vi "SingleFitDoubleExponential.vi"(0 "Scan rate (Hz)":dbl, 5 "Last point to average for baseline":i32=5, 9 "Input decay":dbl[](array[numeric]), 11 "Input Variance":dbl[](array[numeric])) -> (3 "mean and fit":dbl[][](graph), 4 "amplitude":dbl=1.3790672561842066 caption="Amplitude (au)" format="%#_3g", 6 "Standard error Amplitude":dbl=8.774972224805227 format="%#_3g", 8 "Area (au)":dbl=8.774972224805227 format="%#_3g", 10 "Residu (au)":dbl=8.774972224805227 format="%#_3g", 14 "Standard error Tau (us)":dbl=8.774972224805227 format="%#_3g", 15 "Tau (us)":dbl=8.774972224805227 format="%#_3g")   [LabVIEW 2013]
uses:
  <vilib>/Analysis/baseanly.llb/Mean (DBL).vi
  <vilib>/gmath/NumericalOptimization/Nonlinear Curve Fit LM formula string.vi
  <vilib>/gmath/NI_Gmath.lvlib
  <vilib>/Analysis/NI_AALBase.lvlib
panel:
  out "stdev a1":dbl
  out "a1":dbl
  out "Input DecaySize":dbl
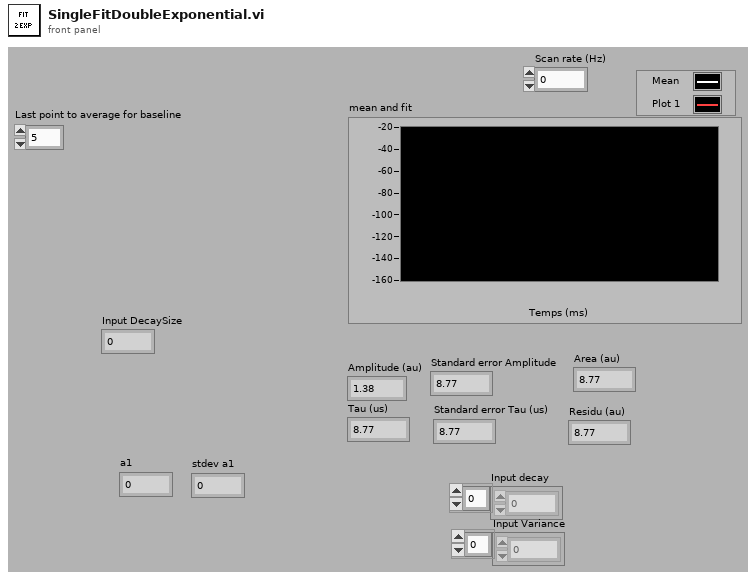
[diagram p1: front panel]
types:
  T1 = cluster{"model":string, "Parameters":string[], "x":string}
  T2 = typedef "NI_Matrix.lvlib/RealMatrix.ctl" = dbl[][]
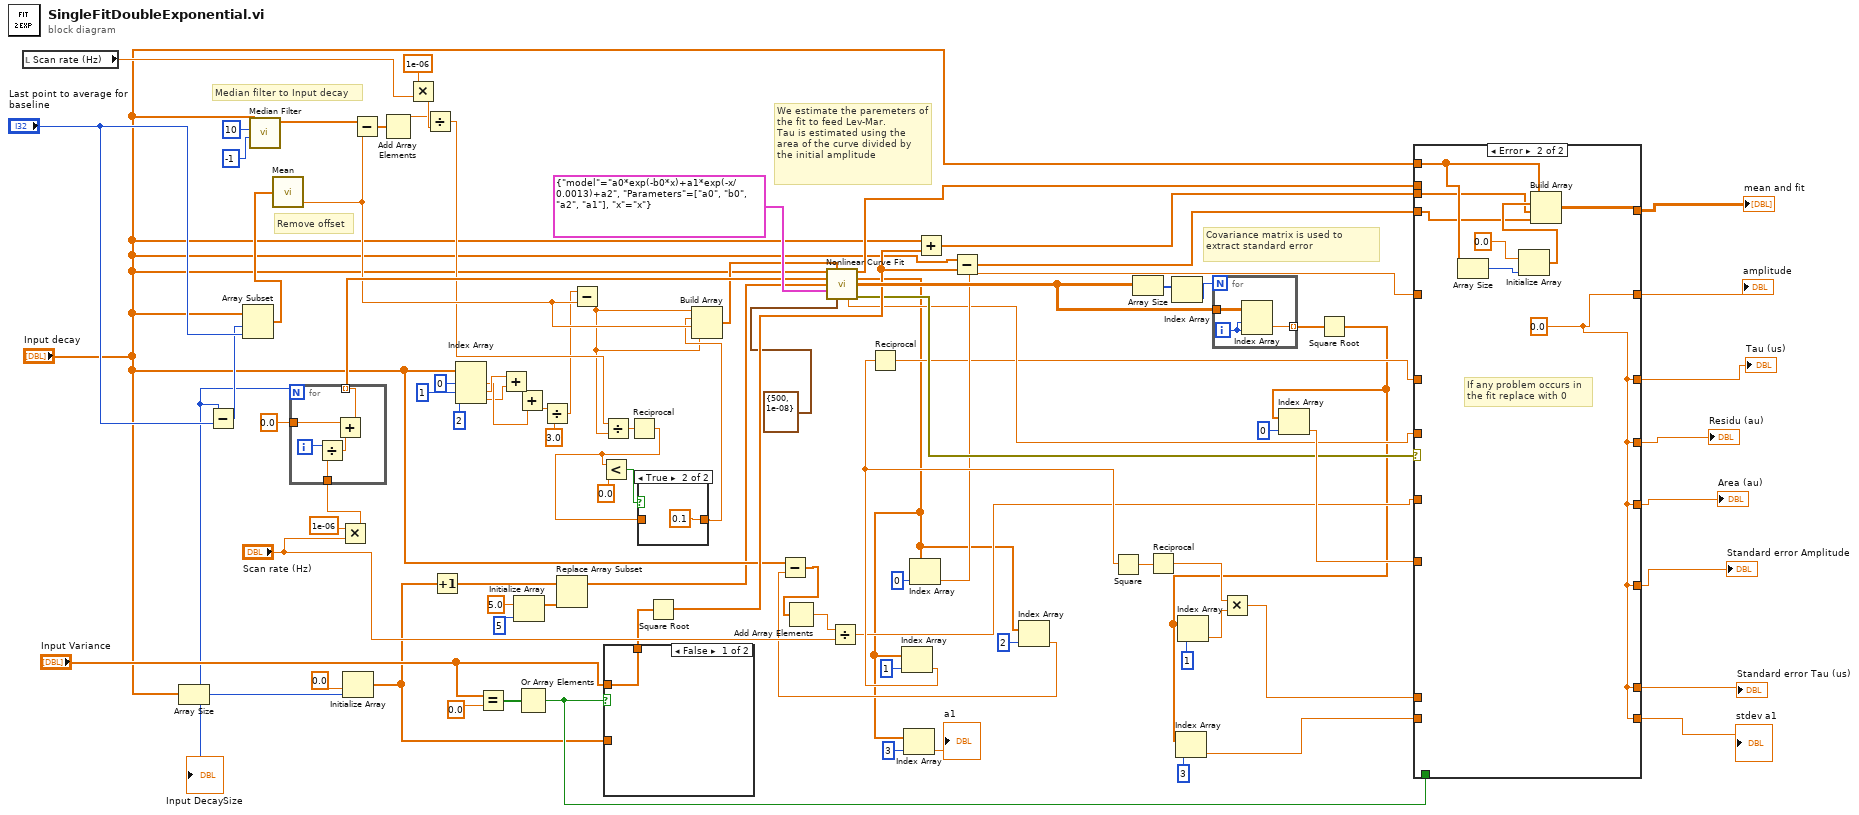
[diagram p0: block diagram]
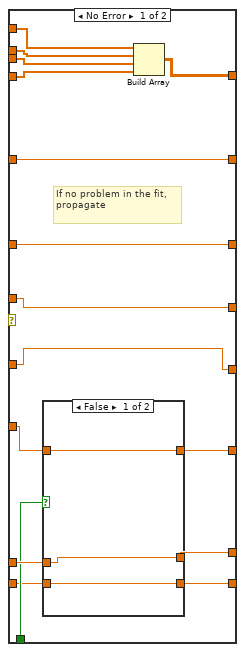
[diagram p3: hidden frame]
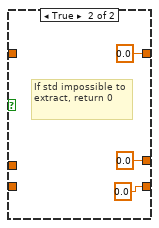
[diagram p4: hidden frame]
diagram:
  # "Median filter to Input decay"
  # "Covariance matrix is used to extract standard error"
  # "Remove offset"
  # "We estimate the paremeters of the fit to feed Lev-Mar.\nTau is estimated using the area of the curve divided by the initial amplitude"
  n1 = local read "Scan rate (Hz)"() -> (w76:dbl)
  n2 = Array Size(array="Input decay") -> (size(s)=w26:i32)
  "Input DecaySize" <- w26
  n3 = Subtract(x=w26, y="Last point to average for baseline") -> (x-y=w91:i32)
  n4 = Array Subset(array="Input decay", index=w91, length="Last point to average for baseline") -> (w90:dbl[])
  n5 = call <vilib>:"Median Filter.vi"("right rank"=-1, "left rank"=10, "X"="Input decay") -> ("Filtered X"=w20:dbl[])  [unwired: 8 out]
  n6 = call-poly <vilib>:"Mean.vi"("X"=w90) -> ("mean"=w36:dbl)  [unwired: 1 out]
  n7 = Multiply(x=1e-06, y="Scan rate (Hz)") -> (x*y=w81:dbl)
  n8 = for {
    N: w26 -> [_]
    tunnel: [w94] -> w83 mode=indexing
    tunnel: w81 -> [w96]
    tunnel: 0.0 -> [w95]
    i -> [w97]
    n9 = Divide(x=w97, y=w96) -> (x/y=w93:dbl)
    n10 = Add(x=w95, y=w93) -> (x+y=w94:dbl)
  }
  n11 = Initialize Array(0.0 ("élément"), w26) -> (w3:dbl[])
  n12 = Subtract(x=w20, y=w36) -> (x-y=w11:dbl[])
  n13 = Add Array Elements(numeric array=w11) -> (sum=w9:dbl)
  n14 = Multiply(x=1e-06, y=w76) -> (x*y=w10:dbl)
  n15 = Divide(x=w9, y=w10) -> (x/y=w27:dbl)
  n16 = Increment(x=w3) -> (x+1=w2:dbl[])
  n17 = Index Array(array="Input decay", index #1=0 ("indice"), index #2=1 ("indice"), index #3=2 ("indice")) -> (element #1=w24:dbl, element #2=w25:dbl, element #3=w23:dbl)
  n18 = Equal?(x="Input Variance", y=0.0 ("élément")) -> (x = y?=w62:bool[])
  n19 = Add(x=w25, y=w23) -> (x+y=w40:dbl)
  n20 = Initialize Array(5.0 ("element"), 5 ("dimension size")) -> (w4:dbl[])
  n21 = Add(x=w40, y=w24) -> (x+y=w38:dbl)
  n22 = Or Array Elements(Boolean array=w62) -> (logical OR=w7:bool)
  n23 = Divide(x=w38, y=3.0) -> (x/y=w22:dbl)
  n24 = Replace Array Subset(array=w2, new element=w4) -> (w1:dbl[])  [unwired: 1 in]
  n25 = Subtract(x=w22, y=w36) -> (x-y=w8:dbl)
  n26 = Divide(x=w27, y=w8) -> (x/y=w39:dbl)
  n27 = case shown="False" w7 {
    tunnel: "Input Variance" -> [w98 _]
    tunnel: w3 -> [_ w99]
    tunnel: [w98 w99] -> w61
    frame False {
    }
    frame True {
      # "If variance is null, remove variance input to Lev-Mar"
    }
  }
  n28 = Reciprocal(x=w39) -> (1/x=w31:dbl)
  n29 = Less?(x=w31, y=0.0) -> (x < y?=w32:bool)
  n30 = case shown="True" w32 {
    tunnel: w31 -> [w100 _]
    tunnel: [w100 0.1] -> w19
    frame False {
    }
    frame True {
    }
  }
  n31 = Square Root(x=w61) -> (sqrt(x)=w57:dbl[])
  n32 = Build Array(w8, w19, w36, w8) -> (w75:dbl[])
  n33 = call-poly <vilib>:"Nonlinear Curve Fit.vi"("Y"="Input decay", "initial parameters"=w75, "X"=w83, "Weight"=w1, "model description"=T1 {"model"="a0*exp(-b0*x)+a1*exp(-x/0.0013)+a2", "Parameters"=["a0", "b0", "a2", "a1"], "x"="x"}, "termination"=cluster{"max iteration":i32, "tolerance":dbl} {"max iteration"=500, "tolerance"=1e-08}) -> ("best nonlinear fit"=w48:dbl[], "best fit parameters"=w17:dbl[], "covariance"=w71:T2, "residue"=w52:dbl, "error out"=w56:errorcluster)  [unwired: 1 in, 4 out]
  n34 = Index Array(array=w17, index=1 ("indice")) -> (element=w64:dbl)
  n35 = Reciprocal(x=w64) -> (1/x=w44:dbl)
  n36 = Index Array(array=w17, index=3) -> (element=→"a1":dbl)
  n37 = Index Array(array=w17, index=0 ("indice")) -> (element=w55:dbl)
  n38 = Add(x="Input decay", y=w57) -> (x+y=w47:dbl[])
  n39 = Subtract(x="Input decay", y=w57) -> (x-y=w46:dbl[])
  n40 = Index Array(array=w17, index=2 ("indice")) -> (element=w74:dbl)
  n41 = Subtract(x="Input decay", y=w74) -> (x-y=w82:dbl[])
  n42 = Add Array Elements(numeric array=w82) -> (sum=w89:dbl)
  n43 = Divide(x=w89, y="Scan rate (Hz)") -> (x/y=w50:dbl)
  n44 = Square(x=w64) -> (x^2=w67:dbl)
  n45 = Array Size(array=w71) -> (size(s)=w73:i32[])
  n46 = Reciprocal(x=w67) -> (1/x=w65:dbl)
  n47 = Index Array(array=w73) -> (element=w72:i32)  [unwired: 1 in]
  n48 = for {
    N: w72 -> [_]
    tunnel: w71 -> [w104]
    tunnel: [w102] -> w70 mode=indexing
    i -> [w103]
    n49 = Index Array(array=w104, index (row)=w103, index (col)=w103) -> (element=w102:dbl)
  }
  n50 = Square Root ("Square Root.vi")(x=w70) -> (sqrt(x)=w14:dbl[])
  n51 = Index Array(array=w14, index=3) -> (element=w12:dbl)
  n52 = Index Array(array=w14, index=1 ("indice")) -> (element=w66:dbl)
  n53 = Multiply(x=w65, y=w66) -> (x*y=w58:dbl)
  n54 = Index Array(array=w14, index=0 ("indice")) -> (element=w60:dbl)
  n55 = case shown="Error" w56 {
    tunnel: w60 -> [w120 _]
    tunnel: [w119 w127] -> w28
    tunnel: [w118 w127] -> w59
    tunnel: w58 -> [w117 _]
    tunnel: w7 -> [w116 _]
    tunnel: [w112 w134] -> w45
    tunnel: w55 -> [w115 _]
    tunnel: [w115 w127] -> w54
    tunnel: [w114 w127] -> w53
    tunnel: w44 -> [w114 _]
    tunnel: w52 -> [w113 _]
    tunnel: [w113 w127] -> w51
    tunnel: w50 -> [w107 _]
    tunnel: [w107 w127] -> w49
    tunnel: "Input decay" -> [w111 w131]
    tunnel: w48 -> [w110 _]
    tunnel: w47 -> [w109 w129]
    tunnel: w46 -> [w108 w128]
    tunnel: [w106 w127] -> w13
    tunnel: w12 -> [w105 _]
    frame No Error {
      # "If no problem in the fit, propagate"
      n56 = case shown="False" w116 {
        tunnel: w120 -> [w123 _]
        tunnel: [w123 0.0 ("Real Matrix Element")] -> w119
        tunnel: [w122 0.0] -> w118
        tunnel: w117 -> [w122 _]
        tunnel: [w121 0.0] -> w106
        tunnel: w105 -> [w121 _]
        frame False {
        }
        frame True {
          # "If std impossible to extract, return 0"
        }
      }
      n57 = Build Array(w111, w110, w109, w108) -> (w112:dbl[][])
    }
    frame Error {
      w127 = 0.0 ("Numeric")
      # "If any problem occurs in the fit replace with 0"
      n58 = Array Size(array=w131) -> (size(s)=w133:i32)
      n59 = Initialize Array(0.0 ("élément"), w133) -> (w130:dbl[])
      n60 = Build Array(w131, w130, w129, w128) -> (w134:dbl[][])
    }
  }
  "amplitude" <- w54
  "Tau (us)" <- w53
  "Area (au)" <- w49
  "Residu (au)" <- w51
  "mean and fit" <- w45
  "Standard error Tau (us)" <- w59
  "Standard error Amplitude" <- w28
  "stdev a1" <- w13
